vi "Address setting.vi"(7 "Address Cluster out输入":T1={"SPU"=refnum, "MPM"=[], "Port_Count"=0.0, "MPM_Count"=0.0, "SPU_Resource"=[], "USB_Resource"=[], "MPM_Communicater"="", "MPM_Count"=0.0, "MPM_Address"=[], "MPM_Portnumber"=[], "SPU_DeviveID"="", "MPM_communcation_method"=[], "TSL_sweepstartwave"=0.0, "TSL_sweepstopwave"=0.0, "TSL_Address"="", "TSL_Communicater"="", "TSL"=refnum, "tsl_communcation_method"=3, "TSL_Portnumber"=0.0, "PCU"=refnum, "PCU_Communicater"="", "PCU_Address"="", "PCU_Portnumber"=0.0, "PCU_useing_internal_DAQ"=FALSE, "PCU_communcation_method"=0} {"PCU_communcation_method" items=["GPIB", "C232C", "TCPIP", "USB"]; "tsl_communcation_method" items=["GPIB", "C232C", "TCPIP", "USB"]; "MPM_communcation_method" items=["GPIB", "C232C", "TCPIP", "USB"]}, 8 "错误输入（无错误）":errorcluster caption="error in", 10 "PowerMonitorType":enum16{"DAQ", "MPM_220", "TSL_LOGG"}(ring), 11 "SPU in":refnum<k24>) -> (0 "error out":errorcluster, 1 "Address Cluster out输出":T1={"SPU"=refnum, "MPM"=[], "Port_Count"=0.0, "MPM_Count"=0.0, "SPU_Resource"=[], "USB_Resource"=[], "MPM_Communicater"="", "MPM_Count"=0.0, "MPM_Address"=[], "MPM_Portnumber"=[], "SPU_DeviveID"="", "MPM_communcation_method"=[], "TSL_sweepstartwave"=0.0, "TSL_sweepstopwave"=0.0, "TSL_Address"="", "TSL_Communicater"="", "TSL"=refnum, "tsl_communcation_method"=3, "TSL_Portnumber"=0.0, "PCU"=refnum, "PCU_Communicater"="", "PCU_Address"="", "PCU_Portnumber"=0.0, "PCU_useing_internal_DAQ"=FALSE, "PCU_communcation_method"=0} {"PCU_communcation_method" items=["GPIB", "C232C", "TCPIP", "USB"]; "tsl_communcation_method" items=["GPIB", "C232C", "TCPIP", "USB"]; "MPM_communcation_method" items=["GPIB", "C232C", "TCPIP", "USB"]})   [LabVIEW 2017]
doc: "'----Apply to communication parametere from Instrument setting form"
uses:
  CTL/Address Cluster.ctl
  D:/test/PDLSTS/LV_PDL LvVer17.0/LV_PDL_x86/DLL/InstrumentDLL.dll
  DLL/InstrumentDLL.dll
  Share/Product_PCU.vi
  Share/MPM_PowerMonitorType.vi
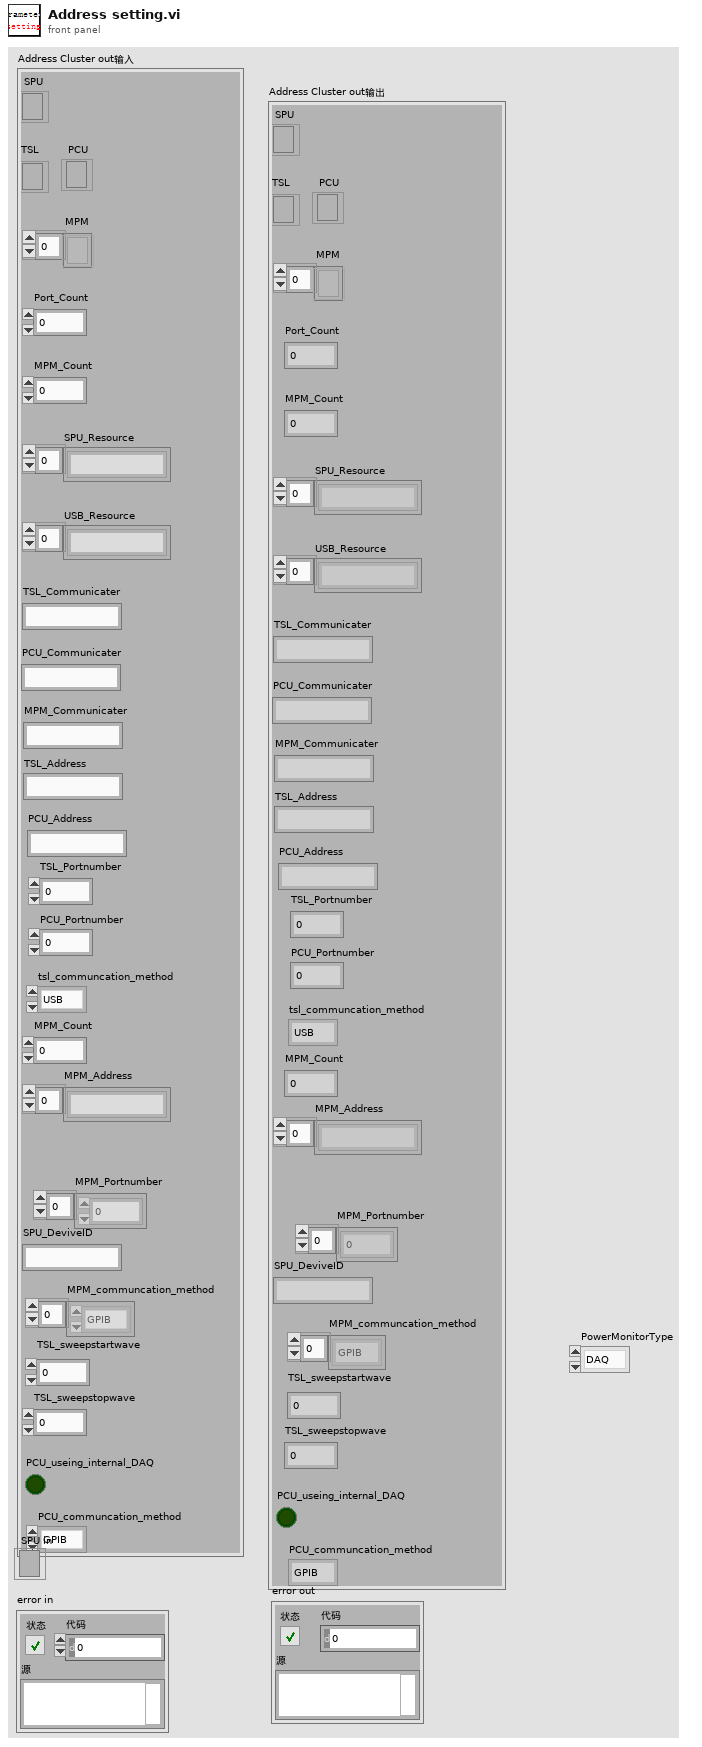
[diagram p1: front panel]
types:
  T1 = typedef "Address Cluster.ctl" = cluster{"SPU":refnum<k24>, "MPM":refnum<k24>[], "Port_Count":dbl, "MPM_Count":dbl, "SPU_Resource":string[], "USB_Resource":string[], "MPM_Communicater":string, "MPM_Count":dbl, "MPM_Address":string[], "MPM_Portnumber":dbl[], "SPU_DeviveID":string, "MPM_communcation_method":i32[], "TSL_sweepstartwave":dbl, "TSL_sweepstopwave":dbl, "TSL_Address":string, "TSL_Communicater":string, "TSL":refnum<k24>, "tsl_communcation_method":i32, "TSL_Portnumber":dbl, "PCU":refnum<k24>, "PCU_Communicater":string, "PCU_Address":string, "PCU_Portnumber":dbl, "PCU_useing_internal_DAQ":bool, "PCU_communcation_method":i32}
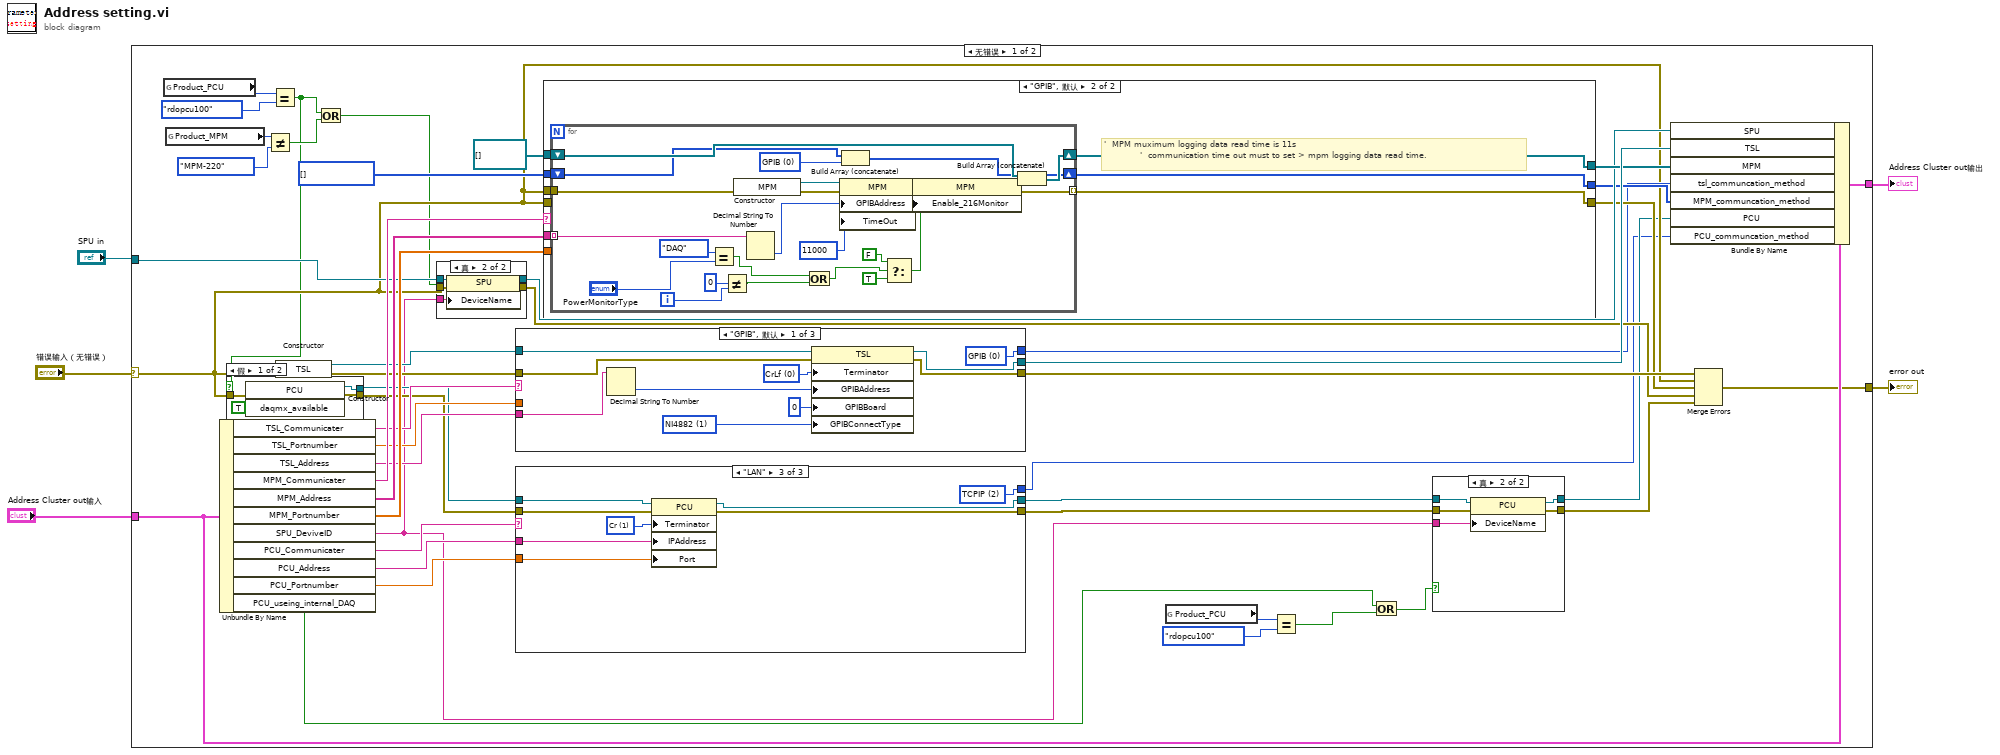
[diagram p0: block diagram]
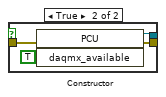
[diagram p2: hidden frame]
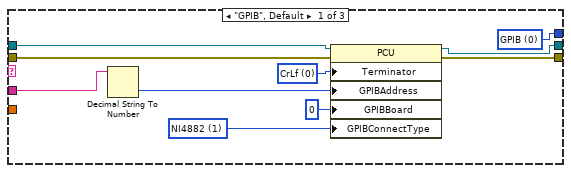
[diagram p5: hidden frame]
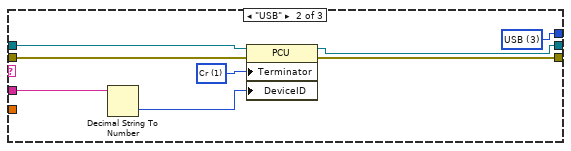
[diagram p6: hidden frame]
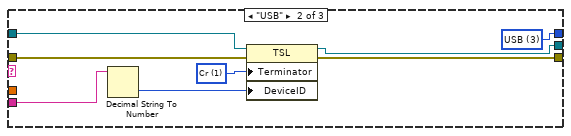
[diagram p7: hidden frame]
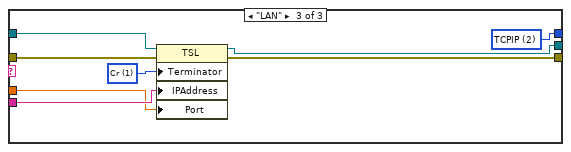
[diagram p8: hidden frame]
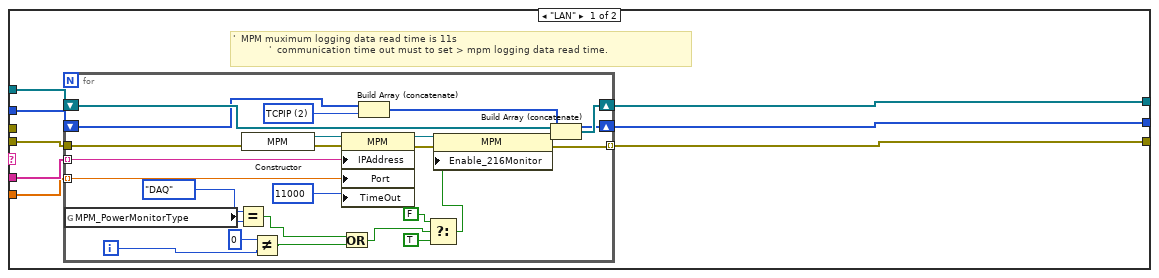
[diagram p9: hidden frame]
diagram:
  n1 = case shown="无错误" "错误输入（无错误）" {
    selector: "错误输入（无错误）" -> [w25 w192]
    tunnel: [w51 w191] -> w5
    tunnel: "Address Cluster out输入" -> [w47 w191]
    tunnel: [w34 w192] -> w3
    tunnel: "SPU in" -> [w33 _]
    frame No Error {
      w46 = i32[] [] items=["GPIB", "C232C", "TCPIP", "USB"] ("tsl_communcation_method")
      n2 = global read "Product_PCU.vi" "Product_PCU"() -> (w11:enum32{"rdopcu100", "rdopcu110"})
      n3 = global read "MPM_PowerMonitorType.vi" "Product_MPM"() -> (w10:enum32{"MPM-210/210H", "MPM-220"})
      n4 = Unbundle By Name(w47) -> ("TSL_Communicater"=w39:string, "TSL_Portnumber"=w41:dbl, "TSL_Address"=w40:string, "MPM_Communicater"=w42:string, "MPM_Address"=w43:string[], "MPM_Portnumber"=w44:dbl[], "SPU_DeviveID"=w18:string, "PCU_Communicater"=w24:string, "PCU_Address"=w27:string, "PCU_Portnumber"=w26:dbl, "PCU_useing_internal_DAQ"=w14:bool)
      n5 = Not Equal?(x=w10, y=enum32{"MPM-210/210H", "MPM-220"}."MPM-220" ("Product_MPM")) -> (x != y?=w8:bool)
      n6 = Equal?(x=w11, y=enum32{"rdopcu100", "rdopcu110"}."rdopcu100" ("Product_PCU")) -> (x = y?=w6:bool)
      n7 = case shown="假" w6 {
        tunnel: [w52 w59] -> w29
        tunnel: [w53 w58] -> w28
        tunnel: w25 -> [w54 w57]
        frame False {
          n8 = constructor class="PCU"(error in=w54, "daqmx_available"=TRUE) -> (reference out=w52:refnum<k24>, error out=w53:errorcluster)  [unwired: 2 in, 2 out]
        }
        frame True {
          n9 = constructor class="PCU"(error in=w57, "daqmx_available"=TRUE) -> (reference out=w59:refnum<k24>, error out=w58:errorcluster)  [unwired: 2 in, 2 out]
        }
      }
      n10 = constructor class="TSL"(error in=w25) -> (reference out=w32:refnum<k24>, error out=w31:errorcluster)  [unwired: 2 in, 1 out]
      n11 = Or(x=w6, y=w8) -> (x .or. y?=w7:bool)
      n12 = case shown="真" w7 {
        tunnel: [w61 w66] -> w48
        tunnel: [w60 w65] -> w35
        tunnel: w33 -> [w61 w64]
        tunnel: w25 -> [w60 w63]
        tunnel: w18 -> [_ w62]
        frame False {
        }
        frame True {
          n13 = property on="属性节点" class="SPU"(reference=w64, error in=w63, "DeviceName"=w62) -> (reference out=w66:refnum<k24>, error out=w65:errorcluster)
        }
      }
      n14 = case shown="\"GPIB\", 默认" w39 {
        tunnel: w32 -> [w109 w117 w125]
        tunnel: [w100 w110 w118] -> w50
        tunnel: w40 -> [w107 w115 w123]
        tunnel: w41 -> [_ _ w122]
        tunnel: w31 -> [w103 w113 w121]
        tunnel: [w102 w112 w120] -> w37
        tunnel: [w101 w111 w119] -> w30
        frame "GPIB", Default {
          w104 = 1 items=["NIVisa", "NI4882", "KeysightIO"] ("GPIBConnectType")
          w108 = 0 items=["CrLf", "Cr", "Lf"] ("Terminator")
          w101 = 0 items=["GPIB", "C232C", "TCPIP", "USB"] ("method")
          n15 = Decimal String To Number(string=w107) -> (number=w106:i32)  [unwired: 2 in, 1 out]
          n16 = property on="属性节点" class="TSL"(reference=w109, error in=w103, "Terminator"=w108, "GPIBAddress"=w106, "GPIBBoard"=0, "GPIBConnectType"=w104) -> (reference out=w100:refnum<k24>, error out=w102:errorcluster)
        }
        frame "USB" {
          w116 = 1 items=["CrLf", "Cr", "Lf"] ("Terminator")
          w111 = 3 items=["GPIB", "C232C", "TCPIP", "USB"] ("method")
          n17 = Decimal String To Number(string=w115) -> (number=w114:i32)  [unwired: 2 in, 1 out]
          n18 = property on="属性节点" class="TSL"(reference=w117, error in=w113, "Terminator"=w116, "DeviceID"=w114) -> (reference out=w110:refnum<k24>, error out=w112:errorcluster)
        }
        frame "LAN" {
          w124 = 1 items=["CrLf", "Cr", "Lf"] ("Terminator")
          w119 = 2 items=["GPIB", "C232C", "TCPIP", "USB"] ("method")
          n19 = property on="属性节点" class="TSL"(reference=w125, error in=w121, "Terminator"=w124, "IPAddress"=w123, "Port"=w122) -> (reference out=w118:refnum<k24>, error out=w120:errorcluster)
        }
      }
      n20 = case shown="\"LAN\"" w24 {
        tunnel: w29 -> [w83 w91 w99]
        tunnel: [w74 w84 w92] -> w23
        tunnel: w27 -> [w81 w89 w97]
        tunnel: w26 -> [_ _ w96]
        tunnel: w28 -> [w77 w87 w95]
        tunnel: [w76 w86 w94] -> w21
        tunnel: [w75 w85 w93] -> w19
        frame "GPIB", Default {
          w78 = 1 items=["NIVisa", "NI4882", "KeysightIO"] ("GPIBConnectType")
          w82 = 0 items=["CrLf", "Cr", "Lf"] ("Terminator")
          w75 = 0 items=["GPIB", "C232C", "TCPIP", "USB"] ("method")
          n21 = Decimal String To Number(string=w81) -> (number=w80:i32)  [unwired: 2 in, 1 out]
          n22 = property on="属性节点" class="PCU"(reference=w83, error in=w77, "Terminator"=w82, "GPIBAddress"=w80, "GPIBBoard"=0, "GPIBConnectType"=w78) -> (reference out=w74:refnum<k24>, error out=w76:errorcluster)
        }
        frame "USB" {
          w90 = 1 items=["CrLf", "Cr", "Lf"] ("Terminator")
          w85 = 3 items=["GPIB", "C232C", "TCPIP", "USB"] ("method")
          n23 = Decimal String To Number(string=w89) -> (number=w88:i32)  [unwired: 2 in, 1 out]
          n24 = property on="属性节点" class="PCU"(reference=w91, error in=w87, "Terminator"=w90, "DeviceID"=w88) -> (reference out=w84:refnum<k24>, error out=w86:errorcluster)
        }
        frame "LAN" {
          w98 = 1 items=["CrLf", "Cr", "Lf"] ("Terminator")
          w93 = 2 items=["GPIB", "C232C", "TCPIP", "USB"] ("method")
          n25 = property on="属性节点" class="PCU"(reference=w99, error in=w95, "Terminator"=w98, "IPAddress"=w97, "Port"=w96) -> (reference out=w92:refnum<k24>, error out=w94:errorcluster)
        }
      }
      n26 = case shown="\"GPIB\", 默认" w42 {
        tunnel: w43 -> [w133 w165]
        tunnel: w44 -> [w132 _]
        tunnel: refnum<k24>[] [] ("添加的数组") -> [w131 w164]
        tunnel: w46 -> [w130 w163]
        tunnel: [w129 w162] -> w49
        tunnel: [w128 w161] -> w38
        tunnel: [w127 w160] -> w36
        tunnel: w25 -> [_ w159]
        tunnel: w25 -> [w126 _]
        frame "LAN" {
          # "'  MPM muximum logging data read time is 11s\n            '  communication time out must to set > mpm logging data read time."
          n27 = for {
            shift-right: [w155] -> w129
            shift-left: w131 -> [w156]
            tunnel: w133 -> [w158] mode=indexing
            tunnel: w132 -> [w157] mode=indexing
            shift-right: [w152] -> w128
            shift-left: w130 -> [w154]
            tunnel: [w137] -> w127 mode=indexing
            tunnel: w126 -> [w150]
            i -> [w141]
            w153 = 2 items=["GPIB", "C232C", "TCPIP", "USB"] ("method")
            n28 = global read "MPM_PowerMonitorType.vi" "MPM_PowerMonitorType"() -> (w134:enum16{"DAQ", "MPM_220", "TSL_LOGG"})
            n29 = Equal?(x=enum16{"DAQ", "MPM_220", "TSL_LOGG"}."DAQ", y=w134) -> (x = y?=w146:bool)
            n30 = constructor class="MPM"(error in=w150) -> (reference out=w149:refnum<k24>, error out=w148:errorcluster)  [unwired: 2 in, 1 out]
            n31 = Not Equal?(x=0, y=w141) -> (x != y?=w145:bool)
            n32 = property on="属性节点" class="MPM"(reference=w149, error in=w148, "IPAddress"=w158, "Port"=w157, "TimeOut"=11000) -> (reference out=w140:refnum<k24>, error out=w139:errorcluster)
            n33 = Or(x=w146, y=w145) -> (x .or. y?=w147:bool)
            n34 = Build Array (concatenate)(w154, w153) -> (w152:i32[])
            n35 = Select(t=FALSE, s=w147, f=TRUE) -> (s? t:f=w136:bool)
            n36 = property on="属性节点" class="MPM"(reference=w140, error in=w139, "Enable_216Monitor"=w136) -> (reference out=w138:refnum<k24>, error out=w137:errorcluster)
            n37 = Build Array (concatenate)(w156, w138) -> (w155:refnum<k24>[])
          }
        }
        frame "GPIB", Default {
          # "'  MPM muximum logging data read time is 11s\n            '  communication time out must to set > mpm logging data read time."
          n38 = for {
            shift-right: [w189] -> w162
            shift-left: w164 -> [w190]
            tunnel: w165 -> [w185] mode=indexing
            shift-right: [w186] -> w161
            shift-left: w163 -> [w188]
            tunnel: [w167] -> w160 mode=indexing
            tunnel: w159 -> [w180]
            i -> [w172]
            w187 = 0 items=["GPIB", "C232C", "TCPIP", "USB"] ("method")
            n39 = Equal?(x=enum16{"DAQ", "MPM_220", "TSL_LOGG"}."DAQ", y="PowerMonitorType") -> (x = y?=w173:bool)
            n40 = Not Equal?(x=0, y=w172) -> (x != y?=w170:bool)
            n41 = constructor class="MPM"(error in=w180) -> (reference out=w182:refnum<k24>, error out=w181:errorcluster)  [unwired: 2 in, 1 out]
            n42 = Decimal String To Number(string=w185) -> (number=w183:i32)  [unwired: 2 in, 1 out]
            n43 = Or(x=w173, y=w170) -> (x .or. y?=w174:bool)
            n44 = property on="属性节点" class="MPM"(reference=w182, error in=w181, "GPIBAddress"=w183, "TimeOut"=11000) -> (reference out=w179:refnum<k24>, error out=w168:errorcluster)
            n45 = Build Array (concatenate)(w188, w187) -> (w186:i32[])
            n46 = Select(t=FALSE, s=w174, f=TRUE) -> (s? t:f=w175:bool)
            n47 = property on="属性节点" class="MPM"(reference=w179, error in=w168, "Enable_216Monitor"=w175) -> (reference out=w169:refnum<k24>, error out=w167:errorcluster)
            n48 = Build Array (concatenate)(w190, w169) -> (w189:refnum<k24>[])
          }
        }
      }
      n49 = global read "Product_PCU.vi" "Product_PCU"() -> (w17:enum32{"rdopcu100", "rdopcu110"})
      n50 = Equal?(x=w17, y=enum32{"rdopcu100", "rdopcu110"}."rdopcu100" ("Product_PCU")) -> (x = y?=w15:bool)
      n51 = Or(x=w14, y=w15) -> (x .or. y?=w13:bool)
      n52 = case shown="真" w13 {
        tunnel: w23 -> [w67 w73]
        tunnel: [w67 w72] -> w22
        tunnel: w21 -> [w68 w71]
        tunnel: [w68 w70] -> w20
        tunnel: w18 -> [_ w69]
        frame False {
        }
        frame True {
          n53 = property class="PCU"(reference=w73, error in=w71, "DeviceName"=w69) -> (reference out=w72:refnum<k24>, error out=w70:errorcluster)
        }
      }
      n54 = Bundle By Name(cluster=w47, "SPU"=w48, "TSL"=w50, "MPM"=w49, "tsl_communcation_method"=w30, "MPM_communcation_method"=w38, "PCU"=w22, "PCU_communcation_method"=w19) -> (w51:T1)
      n55 = Merge Errors(w37, w25, w36, w35, w20) -> (w34:errorcluster)
    }
    frame Error {
    }
  }
  "Address Cluster out输出" <- w5
  "error out" <- w3
